vi "Save defaults.vi"(8 "error in (no error)":errorcluster, 11 "MagLabGraph in":refnum<class "XY Plot.lvclass">) -> (0 "error out":errorcluster, 3 "MagLabGraph out":refnum<class "XY Plot.lvclass">)   [LabVIEW 2015, in "XY Plot.lvclass"]
uses:
  XY Plot.lvclass
  <vilib>/ActorFramework/Actor/Actor.lvclass/Actor.ctl
  XY Plot.lvclass/XY Plot.ctl
  <vilib>/ActorFramework/Actor/Actor.lvclass
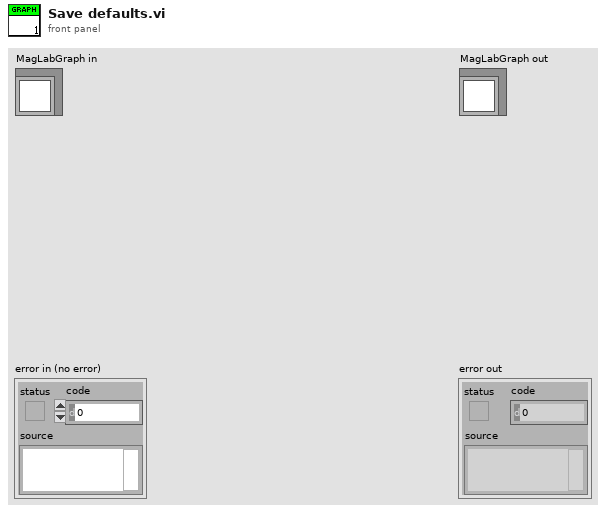
[diagram p1: front panel]
types:
  T1 = cluster{"File Path Control":path, "Group":string, "Channel":string, "Abbreviated":string}[]
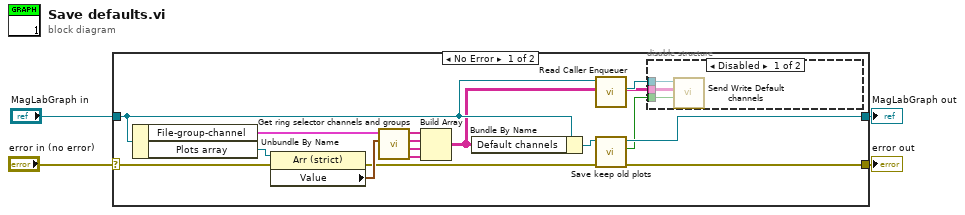
[diagram p0: block diagram]
diagram:
  n1 = case shown="No Error" "error in (no error)" {
    selector: "error in (no error)" -> [w17 w25]
    tunnel: [w9 w25] -> w3
    tunnel: [w11 w24] -> w1
    tunnel: "MagLabGraph in" -> [w8 w24]
    frame No Error {
      n2 = Unbundle By Name(w8) -> ("File-group-channel"=w18:T1, "Plots array"=w20:refnum<vi>)
      n3 = property class="Arr (strict)"(reference=w20, error in=w17) -> (error out=w10:errorcluster, "Value"=w19:cluster{"X":u16, "Y":u16}[])  [unwired: 1 out]
      n4 = call "Get ring selector channels and groups .vi"("Plots  selector"=w19, "File-group-channel"=w18) -> ("Channels Y"=w13:string[], "Groups Y"=w14:string[], "Channels X"=w15:string[], "Groups X"=w16:string[])  [unwired: 6 in]
      n5 = Build Array(w16, w15, w14, w13) -> (w6:string[][])
      n6 = Bundle By Name(cluster=w8, "Default channels"=w6) -> (w12:refnum<class "XY Plot.lvclass">)
      n7 = call <vilib>:"Read Caller Enqueuer.vi"("Actor"=w8) -> ("Caller Enqueuer"=w7:refnum<class "Message Enqueuer.lvclass">)  [unwired: 10 in]
      n8 = call-dynamic "Save keep old plots.vi"("error in (no error)"=w10, "MagLabGraph in"=w12) -> ("error out"=w9:errorcluster, "Value"=w5:bool, "MagLabGraph out"=w11:refnum<class "XY Plot.lvclass">)  [unwired: 7 in]
      n9 = disable-structure shown="Disabled" {
        disable-tunnel: w7 -> [w23 _]
        disable-tunnel: w6 -> [w22 _]
        disable-tunnel: w5 -> [w21 _]
        frame Disabled {
          n10 = call "Send Write Default channels.vi"("Keep old\nplots"=w21, "Default channels"=w22, "Message Enqueuer"=w23) -> ()  [unwired: 7 in, 2 out]
        }
        frame Enabled {
        }
      }
    }
    frame Error {
    }
  }
  "error out" <- w3
  "MagLabGraph out" <- w1
